vi "NVH Outputs Controls Buffer.vi"(8 "Serial Number In":string, 9 "NVH Outputs":bool[](array[boolean]), 10 "NVH Outputs Control":T2[](array[typedef]), 11 "Mode":T1) -> (1 "Serial Number Out":string, 2 "NVH Single Outputs":bool, 3 "NVH Outputs Out":bool[](array[boolean]))   [LabVIEW 2018]
uses:
  02.Type Def's/NVH Digital Output.ctl
  02.Type Def's/NVH Mode Control.ctl
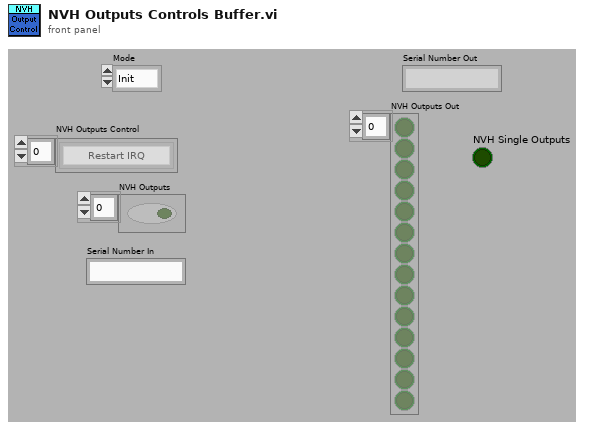
[diagram p1: front panel]
types:
  T1 = typedef "NVH Mode Control.ctl" = enum16{"Init", "Write", "Write String", "Read"}
  T2 = typedef "NVH Digital Output.ctl" = enum16{"Restart IRQ", "Abort Test IRQ", "Read Model", "Start Test", "Stop Test", "End of Test IRQ", "Test Bit 1", "Test Bit 2", "Test Bit 3", "Test Bit 4", "Model Bit 1", "Model Bit 2", "Model Bit 3", "Model Bit 4", "Manual Restart IRQ"}
  T3 = cluster{"B&K Outputs":bool[], "Serial Number":string}
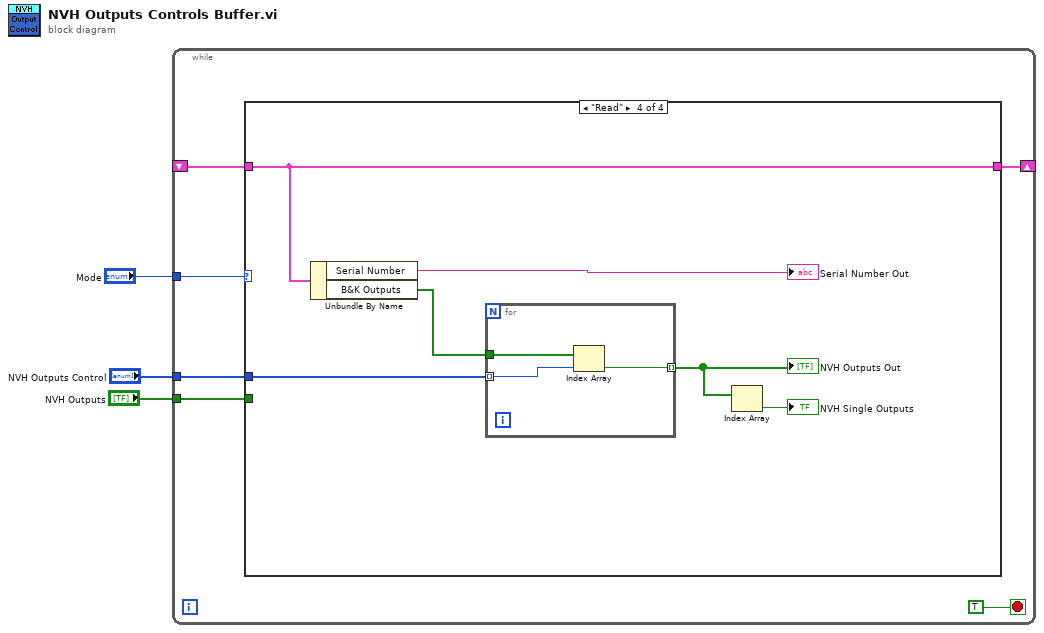
[diagram p0: block diagram]
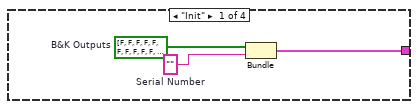
[diagram p2: hidden frame]
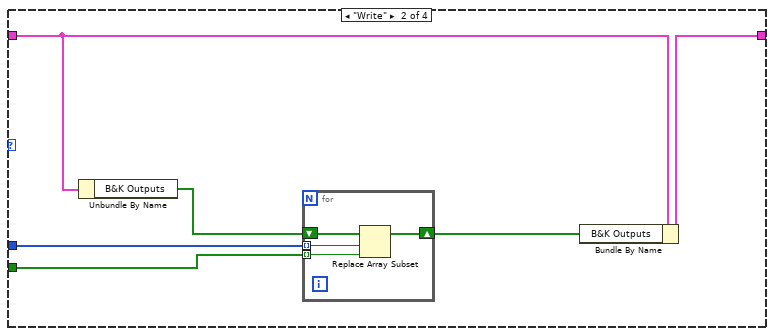
[diagram p3: hidden frame]
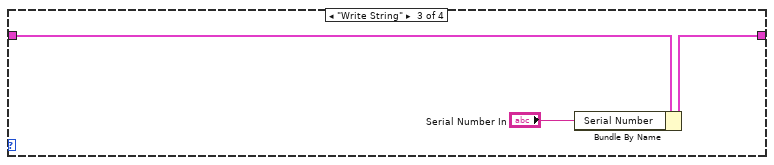
[diagram p4: hidden frame]
diagram:
  n1 = while {
    tunnel: "Mode" -> [w8]
    shift-right: [w6] -> _
    shift-left: _ -> [w7]
    tunnel: "NVH Outputs Control" -> [w5]
    tunnel: "NVH Outputs" -> [w4]
    stop <- TRUE stop-if-true
    n2 = case shown="\"Read\"" w8 {
      tunnel: w7 -> [_ w15 w25 w31]
      tunnel: [w10 w14 w24 w31] -> w6
      tunnel: w5 -> [_ w17 _ w29]
      tunnel: w4 -> [_ w16 _ _]
      frame "Init" {
        w12 = ""  # Serial Number
        w11 = bool[] [FALSE, FALSE, FALSE, FALSE, FALSE, FALSE, FALSE, FALSE, FALSE, FALSE, FALSE, FALSE, FALSE, FALSE, FALSE]  # B&K Outputs
        n3 = Bundle("B&K Outputs"=w11, "Serial Number"=w12) -> (w10:T3)  [unwired: 1 out]
      }
      frame "Write" {
        n4 = Unbundle By Name(w15) -> ("B&K Outputs"=w18:bool[])
        n5 = for {
          shift-right: [w19] -> w13
          shift-left: w18 -> [w22]
          tunnel: w17 -> [w21] mode=indexing
          tunnel: w16 -> [w20] mode=indexing
          n6 = Replace Array Subset(array=w22, new element=w20, index=w21) -> (w19:bool[])
        }
        n7 = Bundle By Name(cluster=w15, "B&K Outputs"=w13) -> (w14:T3)
      }
      frame "Write String" {
        n8 = Bundle By Name(cluster=w25, "Serial Number"="Serial Number In") -> (w24:T3)
      }
      frame "Read" {
        n9 = Unbundle By Name(w31) -> ("Serial Number"=→"Serial Number Out":string, "B&K Outputs"=w28:bool[])
        n10 = for {
          tunnel: w29 -> [w33] mode=indexing
          tunnel: w28 -> [w34]
          tunnel: [w32] -> w27 mode=indexing
          n11 = Index Array(array=w34, index=w33) -> (element=w32:bool)
        }
        "NVH Outputs Out" <- w27
        n12 = Index Array(array=w27) -> (element=→"NVH Single Outputs":bool)  [unwired: 1 in]
      }
    }
  }
